vi "Form GSV Sentence.vi"(8 "error in (no error)":errorcluster, 11 "GSV data":T1={"number of sentences for full data"={"included?"=TRUE, "number of sentences"=0}, "sentence index"={"included?"=TRUE, "index"=0}, "number of satellites in view"={"included?"=TRUE, "number of satellites"=0}, "satellite data"={"included?"=[TRUE, TRUE, TRUE, TRUE], "data"=[]}} {"satellite data"."data"."signal to noise ratio" min=0 max=99; "satellite data"."data"."azimuth (deg)" min=0 max=359; "satellite data"."data"."elevation (deg)" min=0 max=90; "number of satellites in view"."number of satellites" min=0; "sentence index"."index" min=0; "number of sentences for full data"."number of sentences" min=0}) -> (0 "error out":errorcluster, 3 "GSV sentence":string)   [LabVIEW 2017, in "NMEA API.lvlib"]
doc: "Creates an NMEA sentence using the data you specify for a particular sentence type. You must manually select the polymorphic instance to use."
uses:
  <vilib>/robotics/Protocols/NMEA/NMEA API.lvlib
  <vilib>/robotics/Protocols/NMEA/typedefs/GSV Data.ctl
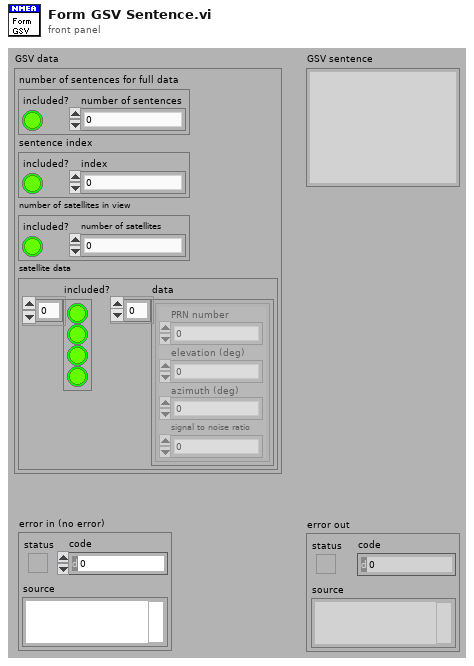
[diagram p1: front panel]
types:
  T1 = typedef "NMEA API.lvlib/GSV Data.ctl" = cluster{"number of sentences for full data":cluster{"included?":bool, "number of sentences":i8}, "sentence index":cluster{"included?":bool, "index":i8}, "number of satellites in view":cluster{"included?":bool, "number of satellites":i8}, "satellite data":cluster{"included?":bool[], "data":cluster{"PRN number":i32, "elevation (deg)":i32, "azimuth (deg)":i32, "signal to noise ratio":i32}[]}}
  T2 = cluster{"included?":bool, "number of sentences":i8}
  T3 = cluster{"included?":bool, "number of satellites":i8}
  T4 = cluster{"included?":bool[], "data":cluster{"PRN number":i32, "elevation (deg)":i32, "azimuth (deg)":i32, "signal to noise ratio":i32}[]}
  T5 = cluster{"PRN number":i32, "elevation (deg)":i32, "azimuth (deg)":i32, "signal to noise ratio":i32}[]
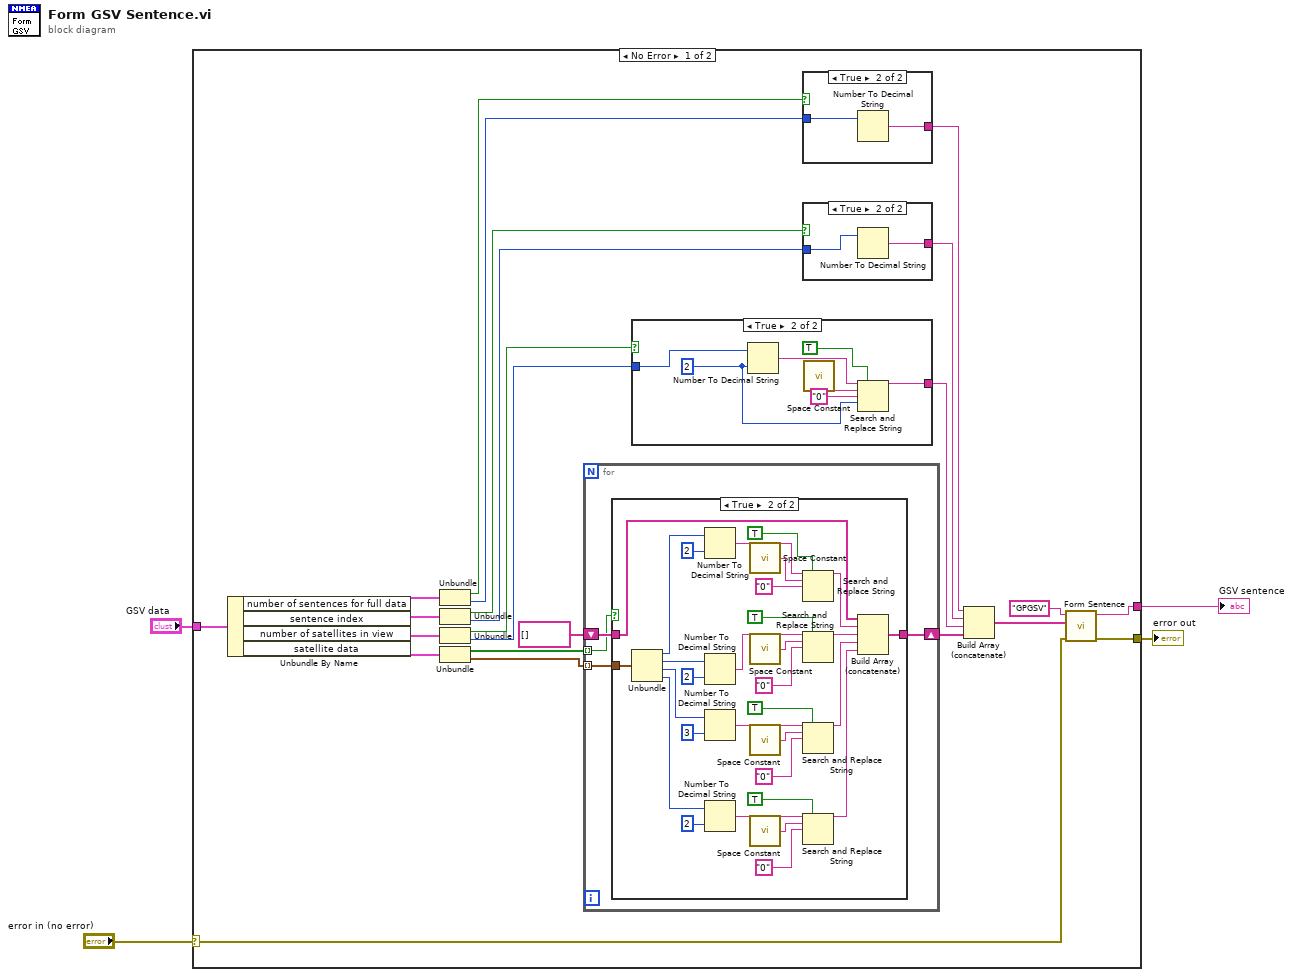
[diagram p0: block diagram]
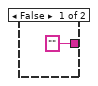
[diagram p3: hidden frame]
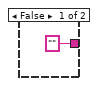
[diagram p4: hidden frame]
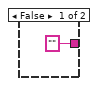
[diagram p5: hidden frame]
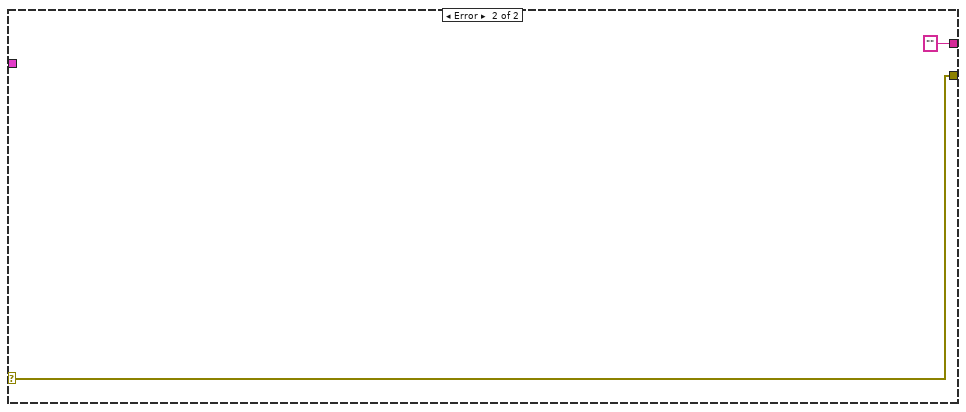
[diagram p6: hidden frame]
diagram:
  n1 = case shown="No Error" "error in (no error)" {
    selector: "error in (no error)" -> [w21 w78]
    tunnel: "GSV data" -> [w27 _]
    tunnel: [w20 w78] -> w2
    tunnel: [w19 "" ("NMEA Sentence")] -> w1
    frame No Error {
      n2 = Unbundle By Name(w27) -> ("number of sentences for full data"=w14:T2, "sentence index"=w13:cluster{"included?":bool, "index":i8}, "number of satellites in view"=w11:T3, "satellite data"=w7:T4)
      n3 = Unbundle(w14) -> ("included?"=w15:bool, "number of sentences"=w16:i8)
      n4 = Unbundle(w13) -> ("included?"=w9:bool, "index"=w12:i8)
      n5 = Unbundle(w11) -> ("included?"=w8:bool, "number of satellites"=w10:i8)
      n6 = Unbundle(w7) -> ("included?"=w5:bool[], "data"=w6:T5)
      n7 = for {
        tunnel: w6 -> [w31] mode=indexing
        shift-right: [w29] -> w17
        shift-left: string[] [] -> [w30]
        tunnel: w5 -> [w28] mode=indexing
        n8 = case shown="True" w28 {
          tunnel: w31 -> [_ w63]
          tunnel: w30 -> [w32 w58]
          tunnel: [w32 w57] -> w29
          frame False {
          }
          frame True {
            n9 = Unbundle(w63) -> ("PRN number"=w62:i32, "elevation (deg)"=w61:i32, "azimuth (deg)"=w60:i32, "signal to noise ratio"=w59:i32)
            n10 = Number To Decimal String(number=w62, width (-)=i16 2) -> (decimal integer string=w54:string)
            n11 = Number To Decimal String(number=w61, width (-)=i16 2) -> (decimal integer string=w46:string)
            n12 = Number To Decimal String(number=w60, width (-)=i16 3) -> (decimal integer string=w40:string)
            n13 = Number To Decimal String(number=w59, width (-)=i16 2) -> (decimal integer string=w34:string)
            n14 = call <vilib>:"Space Constant.vi"() -> ("String"=w53:string)
            n15 = call <vilib>:"Space Constant.vi"() -> ("String"=w48:string)
            n16 = call <vilib>:"Space Constant.vi"() -> ("String"=w42:string)
            n17 = call <vilib>:"Space Constant.vi"() -> ("String"=w36:string)
            n18 = Search and Replace String(replace all?=TRUE ("replace all? (F)"), input string=w54, search string=w53, replace string="0" ("replace string (\"\")")) -> (result string=w51:string)  [unwired: 4 in, 3 out]
            n19 = Search and Replace String(replace all?=TRUE ("replace all? (F)"), input string=w46, search string=w48, replace string="0" ("replace string (\"\")")) -> (result string=w45:string)  [unwired: 4 in, 3 out]
            n20 = Search and Replace String(replace all?=TRUE ("replace all? (F)"), input string=w40, search string=w42, replace string="0" ("replace string (\"\")")) -> (result string=w39:string)  [unwired: 4 in, 3 out]
            n21 = Search and Replace String(replace all?=TRUE ("replace all? (F)"), input string=w34, search string=w36, replace string="0" ("replace string (\"\")")) -> (result string=w33:string)  [unwired: 4 in, 3 out]
            n22 = Build Array (concatenate)(w58, w51, w45, w39, w33) -> (w57:string[])
          }
        }
      }
      n23 = case shown="True" w8 {
        tunnel: ["" w66] -> w24
        tunnel: w10 -> [_ w71]
        frame False {
        }
        frame True {
          w68 = i16 2 ("width (-)")
          n24 = Number To Decimal String(number=w71, width (-)=w68) -> (decimal integer string=w67:string)
          n25 = call <vilib>:"Space Constant.vi"() -> ("String"=w65:string)
          n26 = Search and Replace String(replace all?=TRUE ("replace all? (F)"), input string=w67, search string=w65, replace string="0" ("replace string (\"\")"), offset=w68) -> (result string=w66:string)  [unwired: 3 in, 3 out]
        }
      }
      n27 = case shown="True" w15 {
        tunnel: ["" w77] -> w26
        tunnel: w16 -> [_ w76]
        frame False {
        }
        frame True {
          n28 = Number To Decimal String(number=w76) -> (decimal integer string=w77:string)  [unwired: 1 out]
        }
      }
      n29 = case shown="True" w9 {
        tunnel: ["" w74] -> w25
        tunnel: w12 -> [_ w73]
        frame False {
        }
        frame True {
          n30 = Number To Decimal String(number=w73) -> (decimal integer string=w74:string)  [unwired: 1 out]
        }
      }
      n31 = Build Array (concatenate)(w26, w25, w24, w17) -> (w22:string[])
      n32 = call <vilib>:"Form Sentence.vi"("error in (no error)"=w21, "sentence data"=w22, "sentence type"="GPGSV" ("Sentence Type")) -> ("error out"=w20:errorcluster, "sentence"=w19:string)  [unwired: 5 in]
    }
    frame Error {
    }
  }
  "error out" <- w2
  "GSV sentence" <- w1
